vi "Write String Parameters to string.vi"(1 "Parameters - string":T1[](array[typedef])) -> (0 "String":string)   [LabVIEW 2020, in "Run Utilities.lvlib" / "Optimiser Cell.lvclass"]
uses:
  Optimiser Cell.lvclass
  Optimise parameter - string.ctl
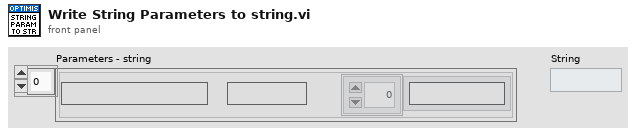
[diagram p1: front panel]
types:
  T1 = typedef "Run Utilities.lvlib/Optimiser Cell.lvclass/Optimise parameter - string.ctl" = cluster{"Name":string, "Start value":string, "Options":string[]}
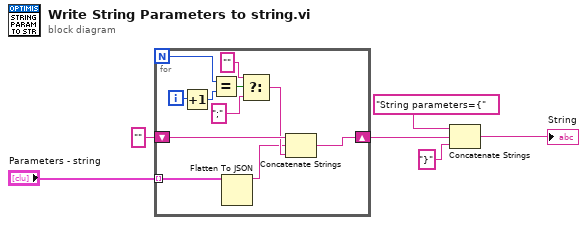
[diagram p0: block diagram]
diagram:
  n1 = for {
    N -> [w13]
    tunnel: "Parameters - string" -> [w8] mode=indexing
    shift-right: [w16] -> w2
    shift-left: "" -> [w17]
    i -> [w15]
    n2 = Increment(x=w15) -> (x+1=w14:i32)
    n3 = Equal?(x=w13, y=w14) -> (x = y?=w12:bool)
    n4 = Flatten To JSON(anything=w8) -> (JSON string=w7:string)  [unwired: 2 in, 1 out]
    n5 = Select(t="" ("string"), s=w12, f=";") -> (s? t:f=w9:string)
    n6 = Concatenate Strings(w17, w7, w9) -> (w16:string)
  }
  n7 = Concatenate Strings("String parameters={" ("string"), w2, "}" ("string")) -> (→"String":string)
